vi "SVT Vibration Level (N Ch).vi"(0 "scaled signals [EU]":waveform(dbl)[](array[waveform]), 1 "integration time [s]":dbl=1.0 format="%.2f", 5 "measurement selection":T1={"RMS"=TRUE, "Running RMS"=FALSE, "Exponential"=FALSE, "Peak"=FALSE, "Max-Min"=FALSE}, 7 "exponential mode":enum16{"Slow", "Fast", "Impulse", "Custom"}(ring)=enum."Fast", 9 "time constant [ms]":dbl=125.0 format="%.2f", 11 "error in (no error)":errorcluster, 12 "restart averaging (F)":bool) -> (3 "exp avg levels [EU rms]":waveform(dbl)[](array[waveform]), 4 "RMS levels [EU rms]":waveform(dbl)[](array[waveform]), 6 "running RMS levels [EU rms]":waveform(dbl)[](array[waveform]), 8 "peak levels [EU]":waveform(dbl)[](array[waveform]), 10 "max-min levels [EU]":waveform(dbl)[](array[waveform]), 14 "unit labels":string[](array[string]), 15 "error out":errorcluster)   [LabVIEW 2017, in "SoundVib_VibrationLevel.lvlib"]
doc: "Computes several vibration level measurements including the root-mean-square (RMS) level, running RMS level, exponential averaged level, peak level, and max-min level. Each instance of this VI maintains its own state; use the N Channel instance of this VI to process an array of channels. This VI operates on time-continuous data; it resets on a discontinuity.<B> Scaled signal [EU]</B> should have a zero DC component. You can attenuate the DC component with hardware AC-coupling filters and with software high-pass filters. Wire data to the <B> scaled signal [EU]</B> input to determine the polymorphic instance to use or manually select the instance."
uses:
  <vilib>/addons/Sound and Vibration/svt_Level/SoundVib_VibrationLevel.lvlib
  <vilib>/addons/Sound and Vibration/svt_Level/SVL Max-Min Level (N Ch).vi
  <vilib>/addons/Sound and Vibration/svt_Level/SVL Peak Level (N Ch).vi
  <vilib>/addons/Sound and Vibration/svt_Level/SVL Decimated Exp Avg Level (N Ch).vi
  <vilib>/addons/Sound and Vibration/svt_Level/SVL Running RMS Level (N Ch).vi
  <vilib>/addons/Sound and Vibration/svt_Level/SVL RMS Level (N Ch).vi
  <vilib>/addons/_NISVFA/_Shared subVIs/Common/svc_Engineering Units to Unit Label.vi
  <vilib>/addons/_NISVFA/_Shared subVIs/Common/svc_Unit Label to Engineering Units.vi
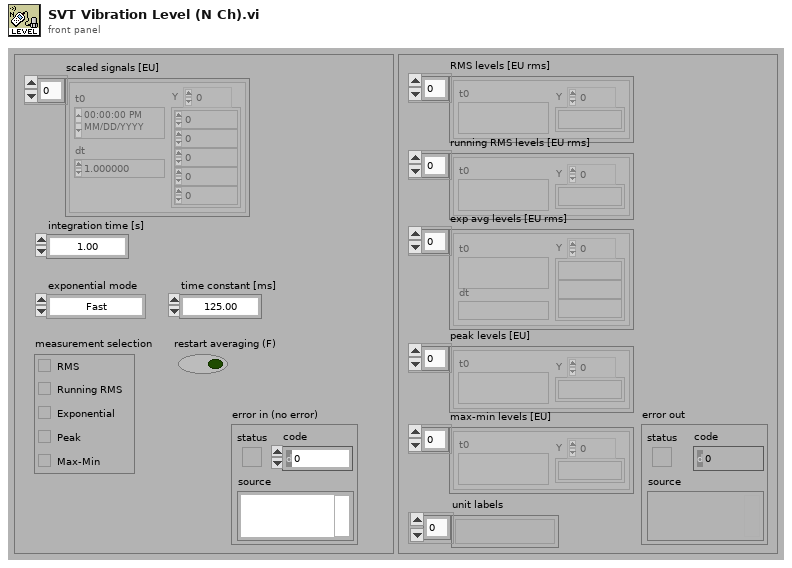
[diagram p1: front panel]
types:
  T1 = cluster{"RMS":bool, "Running RMS":bool, "Exponential":bool, "Peak":bool, "Max-Min":bool}
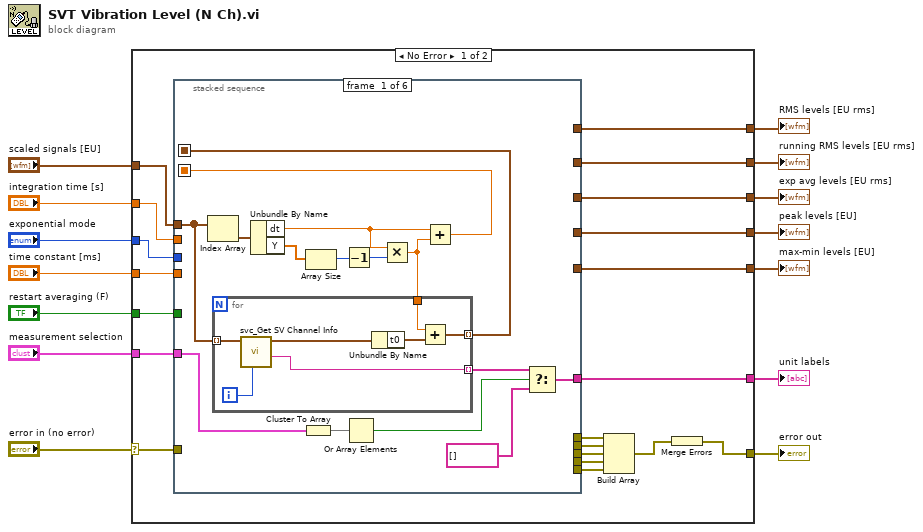
[diagram p0: block diagram]
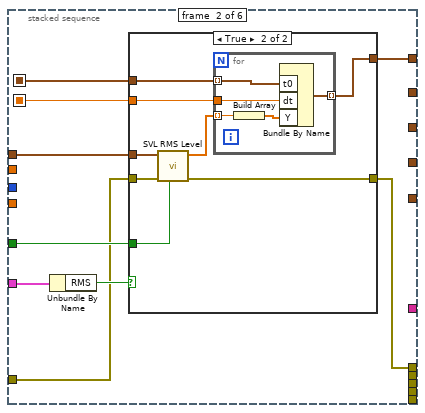
[diagram p2: hidden frame]
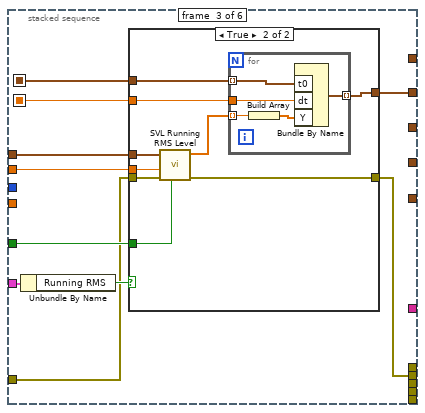
[diagram p4: hidden frame]
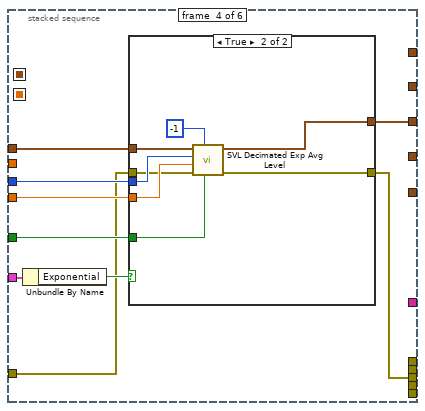
[diagram p6: hidden frame]
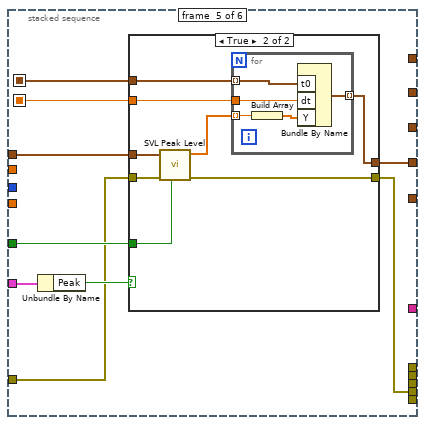
[diagram p8: hidden frame]
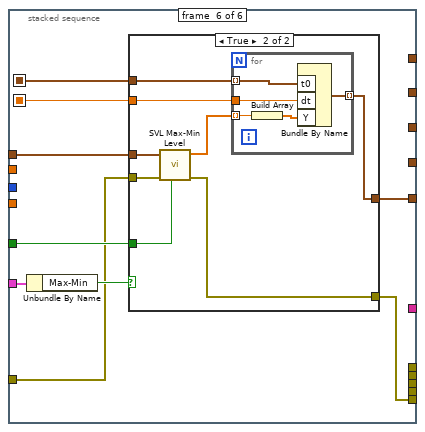
[diagram p10: hidden frame]
diagram:
  n1 = case shown="No Error" "error in (no error)" {
    selector: "error in (no error)" -> [w18 w169]
    tunnel: "scaled signals [EU]" -> [w34 _]
    tunnel: "restart averaging (F)" -> [w33 _]
    tunnel: [w32 _] -> w5
    tunnel: [w31 _] -> w4
    tunnel: "integration time [s]" -> [w30 _]
    tunnel: "exponential mode" -> [w29 _]
    tunnel: "time constant [ms]" -> [w28 _]
    tunnel: [w27 _] -> w3
    tunnel: [w26 _] -> w2
    tunnel: "measurement selection" -> [w25 _]
    tunnel: [w15 _] -> w9
    tunnel: [w19 w169] -> w8
    tunnel: [w16 _] -> w1
    frame No Error {
      n2 = stacked-sequence {
        seq-local: [w46 _ _ _ _ _] -> [_ w60 w84 _ w126 w149]
        seq-local: [w45 _ _ _ _ _] -> [_ w61 w85 _ w127 w150]
        tunnel: w25 -> [w39 w65 w89 w113 w131 w154]
        tunnel: w34 -> [w44 w63 w87 w111 w129 w152]
        tunnel: w33 -> [_ w62 w86 w110 w128 w151]
        tunnel: [_ w59 _ _ _ _] -> w32
        tunnel: [_ _ w83 _ _ _] -> w31
        tunnel: w30 -> [_ _ w82 _ _ _]
        tunnel: w29 -> [_ _ _ w109 _ _]
        tunnel: w28 -> [_ _ _ w108 _ _]
        tunnel: [_ _ _ w107 _ _] -> w27
        tunnel: [_ _ _ _ w125 _] -> w26
        tunnel: w18 -> [_ w58 w81 w106 w124 w148]
        tunnel: [_ w57 _ _ _ _] -> w24
        tunnel: [_ _ w80 _ _ _] -> w23
        tunnel: [_ _ _ w105 _ _] -> w22
        tunnel: [_ _ _ _ w123 _] -> w21
        tunnel: [_ _ _ _ _ w147] -> w17
        tunnel: [_ _ _ _ _ w146] -> w16
        tunnel: [w35 _ _ _ _ _] -> w15
        frame #0 {
          n3 = Index Array(array=w44) -> (element=w43:waveform(dbl))  [unwired: 1 in]
          n4 = Unbundle By Name(w43) -> ("dt"=w41:dbl, "Y"=w49:dbl[])
          n5 = Cluster To Array(cluster=w39) -> (array=w40:bool[])
          n6 = Array Size(array=w49) -> (size(s)=w48:i32)
          n7 = Decrement(x=w48) -> (x-1=w47:i32)
          n8 = Or Array Elements(Boolean array=w40) -> (logical OR=w37:bool)
          n9 = Multiply(x=w41, y=w47) -> (x*y=w42:dbl)
          n10 = for {
            tunnel: w44 -> [w53] mode=indexing
            tunnel: w42 -> [w56]
            tunnel: [w54] -> w45 mode=indexing
            tunnel: [w51] -> w38 mode=indexing
            i -> [w50]
            n11 = call <vilib>:"svc_Get SV Channel Info.vi"("channel index"=w50, "scaled signal [EU]"=w53) -> ("unit label"=w51:string, "dup scaled signal [EU]"=w52:waveform(dbl))  [unwired: 4 in, 4 out]
            n12 = Unbundle By Name(w52) -> ("t0"=w55:timestamp)
            n13 = Add(x=w56, y=w55) -> (x+y=w54:timestamp)
          }
          n14 = Add(x=w41, y=w42) -> (x+y=w46:dbl)
          n15 = Select(t=w38, s=w37, f=string[] []) -> (s? t:f=w35:string[])
        }
        frame #1 {
          n16 = Unbundle By Name(w65) -> ("RMS"=w64:bool)
          n17 = case shown="True" w64 {
            tunnel: w63 -> [_ w74]
            tunnel: w62 -> [_ w73]
            tunnel: w61 -> [_ w72]
            tunnel: w60 -> [_ w71]
            tunnel: [_ w70] -> w59
            tunnel: w58 -> [w66 w69]
            tunnel: [w66 w68] -> w57
            frame False {
            }
            frame True {
              n18 = call-poly <vilib>:"SVL RMS Level.vi"("restart averaging (F)"=w73, "error in (no error)"=w69, "scaled signals [EU]"=w74) -> ("error out"=w68:errorcluster, "RMS levels [EU rms]"=w67:dbl[])  [unwired: 6 in, 1 out]
              n19 = for {
                tunnel: w72 -> [w79] mode=indexing
                tunnel: w71 -> [w78]
                tunnel: [w77] -> w70 mode=indexing
                tunnel: w67 -> [w76] mode=indexing
                n20 = Build Array(w76) -> (w75:dbl[])
                n21 = Bundle By Name("t0"=w79, "dt"=w78, "Y"=w75) -> (w77:waveform(dbl))  [unwired: 1 in]
              }
            }
          }
        }
        frame #2 {
          n22 = Unbundle By Name(w89) -> ("Running RMS"=w88:bool)
          n23 = case shown="True" w88 {
            tunnel: w87 -> [_ w99]
            tunnel: w86 -> [_ w98]
            tunnel: w85 -> [_ w91]
            tunnel: w84 -> [_ w92]
            tunnel: [_ w94] -> w83
            tunnel: w82 -> [_ w97]
            tunnel: w81 -> [w90 w96]
            tunnel: [w90 w95] -> w80
            frame False {
            }
            frame True {
              n24 = call-poly <vilib>:"SVL Running RMS Level.vi"("restart averaging (F)"=w98, "error in (no error)"=w96, "integration time [s]"=w97, "scaled signals [EU]"=w99) -> ("error out"=w95:errorcluster, "running RMS levels [EU rms]"=w93:dbl[])  [unwired: 4 in, 2 out]
              n25 = for {
                tunnel: w91 -> [w104] mode=indexing
                tunnel: w92 -> [w103]
                tunnel: [w102] -> w94 mode=indexing
                tunnel: w93 -> [w101] mode=indexing
                n26 = Build Array(w101) -> (w100:dbl[])
                n27 = Bundle By Name("t0"=w104, "dt"=w103, "Y"=w100) -> (w102:waveform(dbl))  [unwired: 1 in]
              }
            }
          }
        }
        frame #3 {
          n28 = Unbundle By Name(w113) -> ("Exponential"=w112:bool)
          n29 = case shown="True" w112 {
            tunnel: w111 -> [_ w122]
            tunnel: w110 -> [_ w121]
            tunnel: w109 -> [_ w120]
            tunnel: w108 -> [_ w119]
            tunnel: [_ w117] -> w107
            tunnel: w106 -> [w114 w116]
            tunnel: [w114 w115] -> w105
            frame False {
            }
            frame True {
              n30 = call-poly <vilib>:"SVL Decimated Exp Avg Level.vi"("restart averaging (F)"=w121, "decimation factor"=-1, "error in (no error)"=w116, "time constant [ms]"=w119, "exponential mode"=w120, "scaled signals [EU]"=w122) -> ("error out"=w115:errorcluster, "decimated exp avg levels [EU rms]"=w117:waveform(dbl)[])  [unwired: 1 in, 3 out]
            }
          }
        }
        frame #4 {
          n31 = Unbundle By Name(w131) -> ("Peak"=w130:bool)
          n32 = case shown="True" w130 {
            tunnel: w129 -> [_ w140]
            tunnel: w128 -> [_ w139]
            tunnel: w127 -> [_ w134]
            tunnel: w126 -> [_ w136]
            tunnel: [_ w133] -> w125
            tunnel: w124 -> [w132 w138]
            tunnel: [w132 w137] -> w123
            frame False {
            }
            frame True {
              n33 = call-poly <vilib>:"SVL Peak Level.vi"("restart averaging (F)"=w139, "error in (no error)"=w138, "scaled signals [EU]"=w140) -> ("error out"=w137:errorcluster, "peak levels [EU]"=w135:dbl[])  [unwired: 6 in, 1 out]
              n34 = for {
                tunnel: w134 -> [w145] mode=indexing
                tunnel: w136 -> [w144]
                tunnel: [w143] -> w133 mode=indexing
                tunnel: w135 -> [w142] mode=indexing
                n35 = Build Array(w142) -> (w141:dbl[])
                n36 = Bundle By Name("t0"=w145, "dt"=w144, "Y"=w141) -> (w143:waveform(dbl))  [unwired: 1 in]
              }
            }
          }
        }
        frame #5 {
          n37 = Unbundle By Name(w154) -> ("Max-Min"=w153:bool)
          n38 = case shown="True" w153 {
            tunnel: w152 -> [_ w163]
            tunnel: w151 -> [_ w162]
            tunnel: w150 -> [_ w157]
            tunnel: w149 -> [_ w159]
            tunnel: [_ w156] -> w146
            tunnel: w148 -> [w155 w161]
            tunnel: [w155 w160] -> w147
            frame False {
            }
            frame True {
              n39 = call-poly <vilib>:"SVL Max-Min Level.vi"("restart averaging (F)"=w162, "error in (no error)"=w161, "scaled signals [EU]"=w163) -> ("error out"=w160:errorcluster, "max-min levels [EU]"=w158:dbl[])  [unwired: 4 in, 3 out]
              n40 = for {
                tunnel: w157 -> [w168] mode=indexing
                tunnel: w159 -> [w167]
                tunnel: [w166] -> w156 mode=indexing
                tunnel: w158 -> [w165] mode=indexing
                n41 = Build Array(w165) -> (w164:dbl[])
                n42 = Bundle By Name("t0"=w168, "dt"=w167, "Y"=w164) -> (w166:waveform(dbl))  [unwired: 1 in]
              }
            }
          }
        }
      }
      n43 = Build Array(w24, w23, w22, w21, w17) -> (w20:errorcluster[])
      n44 = Merge Errors(w20) -> (w19:errorcluster)
    }
    frame Error {
    }
  }
  "error out" <- w8
  "unit labels" <- w9
  "peak levels [EU]" <- w2
  "exp avg levels [EU rms]" <- w3
  "RMS levels [EU rms]" <- w5
  "running RMS levels [EU rms]" <- w4
  "max-min levels [EU]" <- w1
